vi "Initialize SV Interface.vi"(8 "error in (no error)":errorcluster, 11 "Process Data":T2={"Write URLs"={"URLs"=[], "Index DBL"=[], "Index Bool"=[]}, "Read URLs"={"URLs"=[], "Index DBL"=[], "Index Bool"=[]}, "Write SV FIFO"="", "Read SV FIFO"="", "Status Notifier"="", "Update Rate"=10}) -> (0 "error out":errorcluster, 3 "SV Data":T1)   [LabVIEW 2016, in "Shared Variable Interface.lvlib"]
uses:
  Shared Variable Interface.lvlib
  Shared DataTypes/SV Process Data.ctl
  Shared DataTypes/URLs.ctl
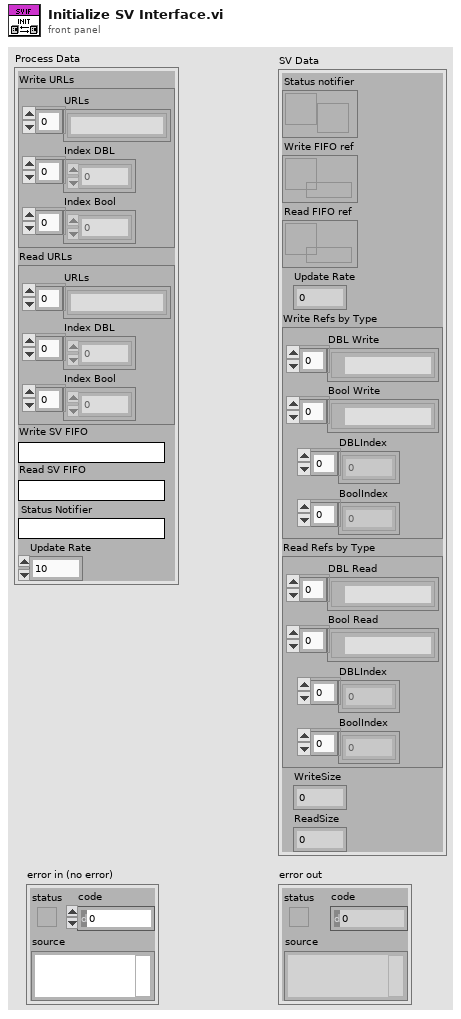
[diagram p1: front panel]
types:
  T1 = cluster{"Status notifier":refnum<notifier>, "Write FIFO ref":refnum<k33>, "Read FIFO ref":refnum<k33>, "Update Rate":u32, "Write Refs by Type":cluster{"DBL Write":refnum<k21>[], "Bool Write":refnum<k21>[], "DBLIndex":i32[], "BoolIndex":i32[]}, "Read Refs by Type":cluster{"DBL Read":refnum<k21>[], "Bool Read":refnum<k21>[], "DBLIndex":i32[], "BoolIndex":i32[]}, "WriteSize":i32, "ReadSize":i32}
  T2 = typedef "SV Process Data.ctl" = cluster{"Write URLs":T3, "Read URLs":T3, "Write SV FIFO":string, "Read SV FIFO":string, "Status Notifier":string, "Update Rate":u32}
  T3 = typedef "URLs.ctl" = cluster{"URLs":string[], "Index DBL":i32[], "Index Bool":i32[]}
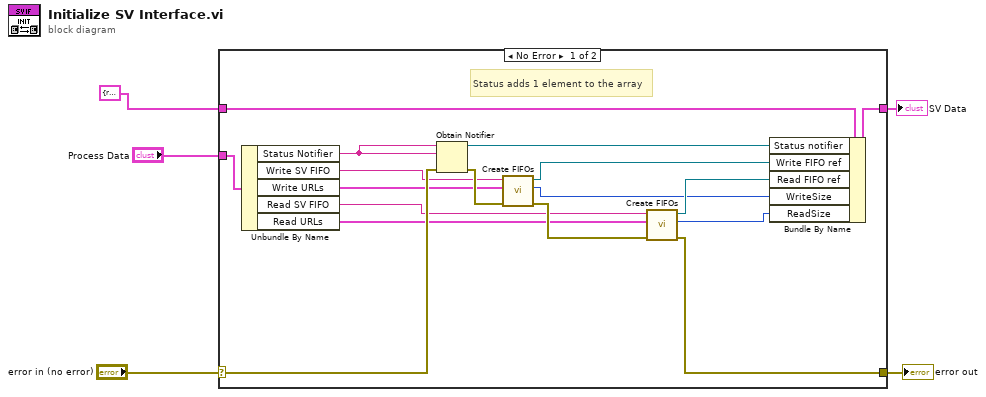
[diagram p0: block diagram]
diagram:
  n1 = case shown="No Error" "error in (no error)" {
    selector: "error in (no error)" -> [w21 w24]
    tunnel: [w13 w24] -> w4
    tunnel: [w18 w23] -> w1
    tunnel: T1 {"Status notifier"=refnum, "Write FIFO ref"=refnum, "Read FIFO ref"=refnum, "Update Rate"=1, "Write Refs by Type"={"DBL Write"=[], "Bool Write"=[], "DBLIndex"=[], "BoolIndex"=[]}, "Read Refs by Type"={"DBL Read"=[], "Bool Read"=[], "DBLIndex"=[], "BoolIndex"=[]}, "WriteSize"=0, "ReadSize"=0} ("SV Data") -> [w19 w23]
    tunnel: "Process Data" -> [w16 _]
    frame No Error {
      # "Status adds 1 element to the array"
      n2 = Unbundle By Name(w16) -> ("Status Notifier"=w22:string, "Write SV FIFO"=w11:string, "Write URLs"=w15:T3, "Read SV FIFO"=w10:string, "Read URLs"=w12:T3)
      n3 = Obtain Notifier(name (unnamed)=w22, notification data type=w22, error in (no error)=w21) -> (notifier out=w17:refnum<notifier>, error out=w20:errorcluster)  [unwired: 1 in, 1 out]
      n4 = call "Create FIFOs.vi"("error in (no error)"=w20, "URL Cluster"=w15, "SV FIFO Name"=w11) -> ("error out"=w14:errorcluster, "size"=w7:i32, "FIFO ref"=w9:refnum<k33>)  [unwired: 6 in]
      n5 = call "Create FIFOs.vi"("error in (no error)"=w14, "URL Cluster"=w12, "SV FIFO Name"=w10) -> ("error out"=w13:errorcluster, "size"=w6:i32, "FIFO ref"=w8:refnum<k33>)  [unwired: 6 in]
      n6 = Bundle By Name(cluster=w19, "Status notifier"=w17, "Write FIFO ref"=w9, "Read FIFO ref"=w8, "WriteSize"=w7, "ReadSize"=w6) -> (w18:T1)
    }
    frame Error {
    }
  }
  "error out" <- w4
  "SV Data" <- w1
